vi "WaitFor2DBufferExample.vi"() -> ()   [LabVIEW 2012]
doc: "A short program to demonstrate the fundamentals of control and image acquision with the pco.camera series. The program records a sequence of images, with \"live\" updating, until the \"StopRecording\" button is pressed. A subset of recorded images is then read out from the camera RAM. Warning: Limit the number of images read back tfrom the camera RAM to a reasonable number. Images are stored as a three-dimensional array, which can very large. Use ctrl-H for more help on the individual controls and indicators.\n\nCopyright 2004, the Cooke Corporation."
panel:
  out "bClose":bool
  in  "Quit":bool
  in  "ImageNr":i32
  in  "Image":i32
  out "BufNr1":i16
  out "BufNr0":i16
  in  "bUseBuffer1":bool
  in  "bUseBuffer0":bool
  in  "ROIX1":u16=1 min=1
  in  "ROIY1":u16=1 min=1
  in  "ROIY0":u16=1 min=1
  in  "ROIX0":u16=1 min=1
  in  "InterfaceType":u16(ring)=5 items=["IEEE1394 - Firewire", "IEEE1394/Firewire", "Matrox Helios Camera Link", "Silicon Software ME3 Camera Link", "National Instruments Camera Link", "Gigabit Ethernet", "USB", "Reserved", "Reserved", "Reserved", "Generic Camera Link with CLSER.DLL"]
  out "Bits/pixel":u16
  in  "Readout":bool
  in  "Record":bool
  in  "Open StructureIn":T1={"Size"=88, "InterfaceType"=0, "Camera Number"=0, "CameraNumAtInterface"=0, "OpenFlags"=[], "OpenDWFlags"=[], "OpenPtrs"=[]}
  in  "Stop":u32=10 min=1
  in  "Start":u32=1 min=1
  in  "DelayTimeBase":u16(ring)=2 items=["nanoseconds", "microseconds", "milliseconds"]
  in  "ExposureTimeBase":u16(ring)=2 items=["nanoseconds", "microseconds", "milliseconds"]
  in  "Exposure":u32=10
  in  "Delay":u32
  out "Reading":bool
  in  "StorageMode":bool
  out "ImageCount":u32
  in  "Rate":i32
  out "Image":u16[][](graph)
  in  "TriggerMode":u16(ring) items=["Auto", "Software", "External sequence start ", "External exposure control"]
  # "A short program to demonstrate the fundamentals of control and image acquision with the pco.camera series. The program records a sequence of images, with \"live\" updating, until the \"StopRecording\" button is pressed. A subset of recorded images is then read out from the camera RAM. WARNING: Limit the number of images read back tfrom the camera RAM to a reasonable number. Images are stored as a three-dimensional array, which can very large.  Use ctrl-H for more help on the individual controls and indicators."
  # "pco.labview"
  # "1) Setup camera:"
  # "FIFO"
  # "Recorder"
  # "2) Record  images:"
  # "3) Read out images:"
  # "4) Display image:"
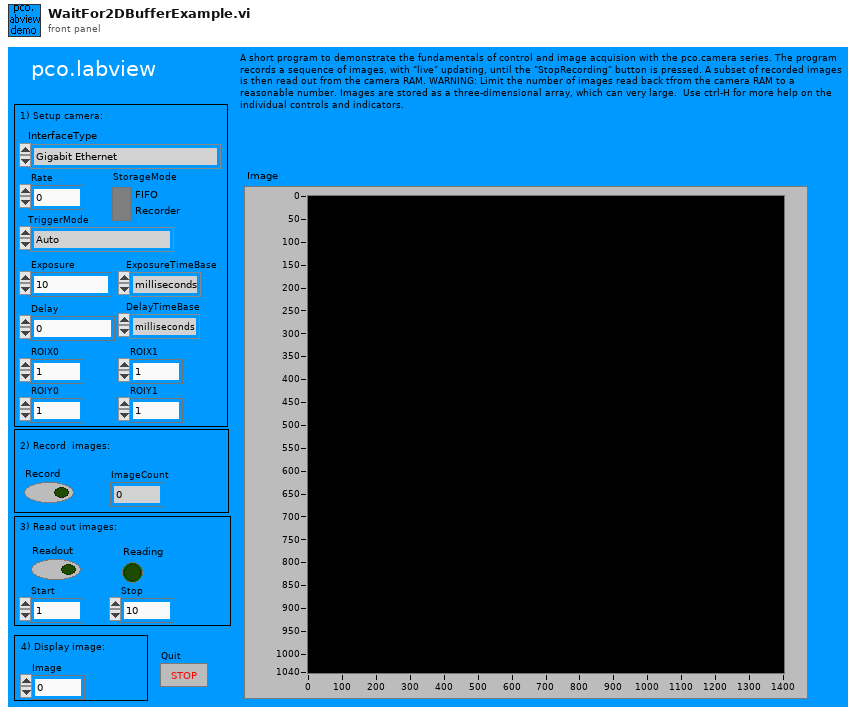
[diagram p1: front panel]
types:
  T1 = cluster{"Size":u16, "InterfaceType":u16, "Camera Number":u16, "CameraNumAtInterface":u16, "OpenFlags":u16[], "OpenDWFlags":u32[], "OpenPtrs":u32[]}
  T2 = cluster{"Size":u16, "CamType":u16, "CamSubType":u16, "SerialNumber":u32, "HWVersion":u32, "FWVersion":u32, "InterfaceType":u16, "HardwareVersion":cluster{"BoardNum":u16, "HWVersions":cluster{"BoardName":string, "BatchNumber":u16, "MinorRevision":u8, "MajorRevision":u8, "Variant":u16}[]}, "FirmwareVersion":cluster{"DeviceNum":u16, "FWVersions":cluster{"DeviceName":string, "MinorRevision":u8, "MajorRevision":u8, "Variant":u16}[]}}
  T3 = cluster{"Size":u16, "SensorTypeDESC":u16, "SensorSubtypeDESC":u16, "MaxHorizontalResStdDESC":u16, "MaxVerticalResStdDESC":u16, "MaxHorizontalResExtDESC":u16, "MaxVerticalResExtDESC":u16, "DynResDESC":u16, "MaxBinHorzDESC":u16, "BinHorzStepDESC":bool, "MaxBinVertDESC":u16, "BinVertStepDESC":bool, "ROIHorzStepDESC":u16, "ROIVertStepDESC":u16, "NumADCDESC":u16, "IRDESC":bool, "MinDelayDESC":u32, "MaxDelayDESC":u32, "MinDelayStepDESC":u32, "MinExpoDESC":u32, "MaxExpoDESC":u32, "MinExpoStepDESC":u32, "MinDelayIRDESC":u32, "MaxDelayIRDESC":u32, "MinExpoIRDESC":u32, "MaxExpoIRDESC":u32, "TimeTableDESC":bool, "DoubleImageDESC":bool, "MinCoolSetDESC":i16, "MaxCoolSetDESC":i16, "MDefaultCoolSetDESC":i16, "PowerDownModeDESC":bool, "OffsetRegDESC":bool, "ColorPattern":cluster{"UpperLeftColor":u8, "UpperRightColor":u8, "LowerLeftColor":u8, "LowerRightColor":u8}, "PatternTypeDESC":bool, "PixelRates":u32[], "CoversionFactors":u16[], "Reserved":u32[], "NoiseFilterCapable":bool, "HotPixelCapable":bool, "HotPixelWithNoiseFilter":bool, "ASCIITimeCapable":bool, "Extended Description":bool, "Get Extended":bool, "Reserved Flag 1":bool, "Reserved Flag 2":bool}
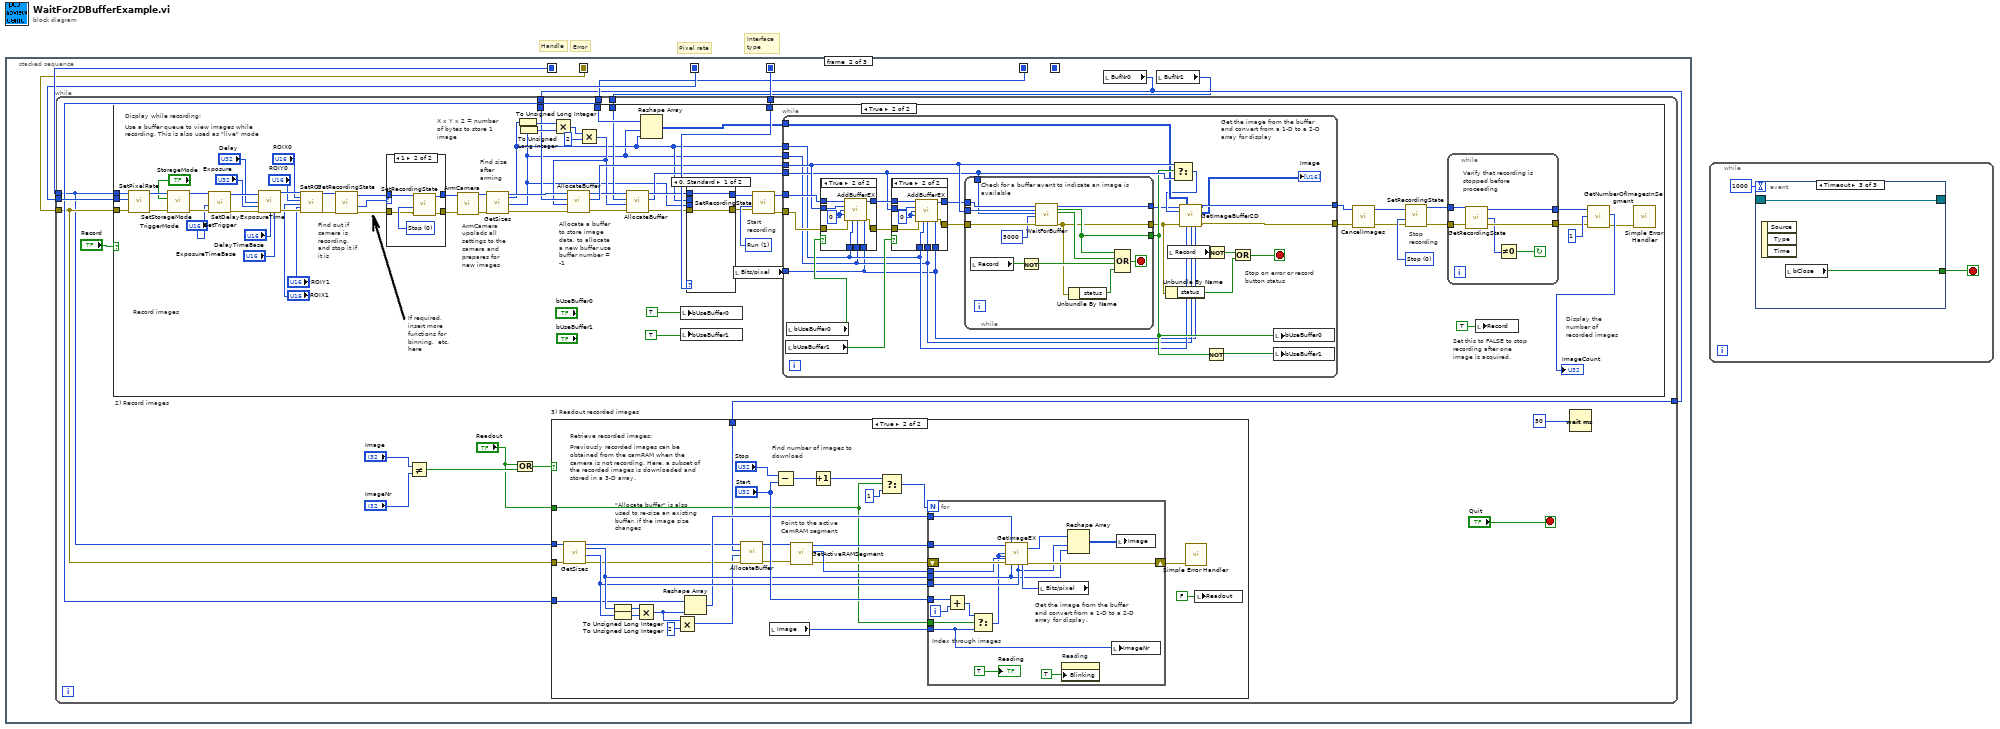
[diagram p0: block diagram]
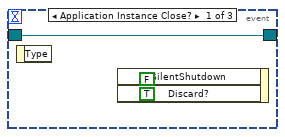
[diagram p2: hidden frame]
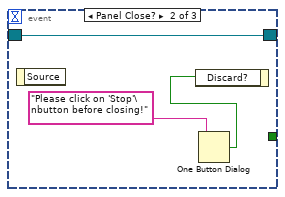
[diagram p3: hidden frame]
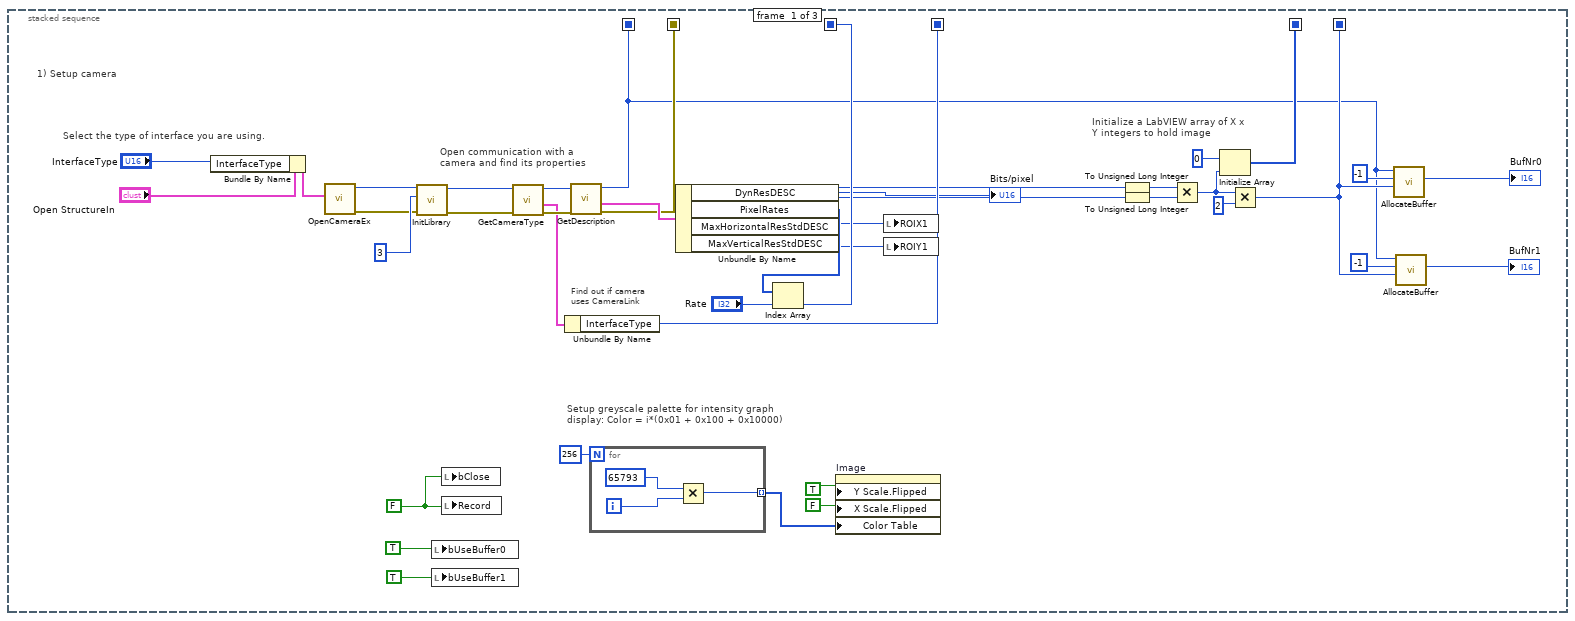
[diagram p4: hidden frame]
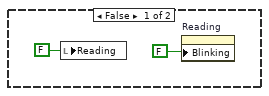
[diagram p5: hidden frame]
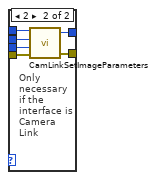
[diagram p9: hidden frame]
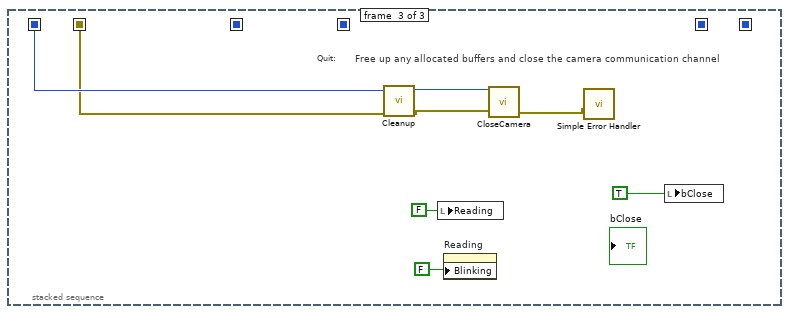
[diagram p11: hidden frame]
diagram:
  # "Interface type"
  # "Error"
  # "Handle"
  # "Pixel rate"
  n1 = stacked-sequence {
    seq-local: [w33 _ _] -> [_ w45 _]
    seq-local: [w13 _ _] -> [_ _ _]
    seq-local: [w25 _ _] -> [_ w47 _]
    seq-local: [w12 _ _] -> [_ w49 w269]
    seq-local: [w24 _ _] -> [_ w48 w268]
    seq-local: [w23 _ _] -> [_ w46 _]
    frame #0 {
      w6 = FALSE ("stop")
      # "Select the type of interface you are using."
      # "1) Setup camera"
      # "Find out if camera uses CameraLink"
      # "Setup greyscale palette for intensity graph display: Color = i*(0x01 + 0x100 + 0x10000)"
      # "Initialize a LabVIEW array of X x Y integers to hold image"
      # "Open communication with a camera and find its properties"
      n2 = Bundle By Name(cluster="Open StructureIn", "InterfaceType"="InterfaceType") -> (w20:T1)
      n3 = call "OpenCameraEx.vi"("OpenStructureIn"=w20) -> ("error out"=w3:errorcluster, "hout"=w4:u64)  [unwired: 3 in, 2 out]
      n4 = call "InitLibrary.vi"("error in (no error)"=w3, "InterfaceType"=u32 3, "ph"=w4) -> ("error out"=w1:errorcluster, "hout"=w2:u64)  [unwired: 7 in]
      n5 = local write "bUseBuffer0"(TRUE) -> ()
      n6 = local write "bUseBuffer1"(TRUE) -> ()
      n7 = local write "bClose"(w6) -> ()
      n8 = local write "Record"(w6) -> ()
      n9 = call "GetCameraType.vi"("ph"=w2, "error in (no error)"=w1) -> ("hout"=w29:u64, "CameraType"=w27:T2, "error out"=w28:errorcluster)  [unwired: 1 in, 1 out]
      n10 = Unbundle By Name(w27) -> ("InterfaceType"=w23:u16)
      n11 = call "GetDescription.vi"("ErrorIn"=w28, "ph"=w29) -> ("ErrorOut"=w24:errorcluster, "Description"=w32:T3, "hout"=w12:u64)  [unwired: 2 in, 1 out]
      n12 = for {
        N: 256 -> [_]
        tunnel: [w40] -> w36 mode=indexing
        i -> [w41]
        n13 = Multiply(x=65793, y=w41) -> (x*y=w40:i32)
      }
      n14 = Unbundle By Name(w32) -> ("DynResDESC"=→"Bits/pixel":u16, "PixelRates"=w26:u32[], "MaxHorizontalResStdDESC"=w18:u16, "MaxVerticalResStdDESC"=w17:u16)
      n15 = Index Array(array=w26, index="Rate") -> (element=w25:u32)
      n16 = property on="Image" class="IntGraph (strikt)"("Y Scale.Flipped"=TRUE, "X Scale.Flipped"=FALSE, "Color Table"=w36) -> ()  [unwired: 2 in, 2 out]
      n17 = local write "ROIX1"(w18) -> ()
      n18 = local write "ROIY1"(w17) -> ()
      n19 = To Unsigned Long Integer(number=w18) -> (unsigned 32bit integer=w15:u32)
      n20 = To Unsigned Long Integer(number=w17) -> (unsigned 32bit integer=w14:u32)
      n21 = Multiply(x=w15, y=w14) -> (x*y=w34:u32)
      n22 = Initialize Array(u16 0 ("Element Data"), w34) -> (w33:u16[])
      n23 = Multiply(x=w34, y=u32 2) -> (x*y=w13:u32)
      n24 = call "AllocateBuffer.vi"("Size"=w13, "BufNr"=i16 -1, "ph"=w12) -> ("BufNrOut"=→"BufNr0":i16)  [unwired: 3 in, 5 out]
      n25 = call "AllocateBuffer.vi"("Size"=w13, "BufNr"=-1, "ph"=w12) -> ("BufNrOut"=→"BufNr1":i16)  [unwired: 3 in, 5 out]
    }
    frame #1 {
      n26 = local read "BufNr0"() -> (w44:i16)
      n27 = local read "BufNr1"() -> (w43:i16)
      n28 = while {
        tunnel: w44 -> [w58]
        tunnel: w44 -> [w59]
        tunnel: w45 -> [w61]
        tunnel: w46 -> [w62]
        tunnel: w47 -> [w63]
        tunnel: w48 -> [w60]
        tunnel: w49 -> [w56]
        tunnel: w43 -> [w57]
        stop <- "Quit" stop-if-true
        n29 = case "2) Record images" shown="True" "Record" {
          tunnel: w56 -> [_ w158]
          tunnel: w60 -> [_ w157]
          tunnel: w63 -> [_ w155]
          tunnel: w62 -> [_ w154]
          tunnel: w61 -> [_ w152]
          tunnel: w59 -> [_ w137]
          tunnel: w57 -> [_ w131]
          frame False {
          }
          frame True {
            w182 = u16 1 items=["Stop", "Run"] ("RecordingState")
            w185 = u16 0 items=["Stop", "Run"] ("RecordingState")
            # "Set this to FALSE to stop recording after one image is acquired."
            # "Display the number of recorded images"
            # "Record images"
            # "Start recording"
            # "Allocate a buffer to store image data. to allocate a new buffer use buffer number = -1"
            # "Find size after arming"
            # "ArmCamera upolads all settings to the camera and prepares for new images"
            # "Find out if camera is recording, and stop it if it is"
            # "If required, insert more functions for binning.  etc. here"
            # "X x Y x 2 = number of bytes to store 1 image"
            # "Stop recording"
            # "Use a buffer queue to view images while recording. This is also used as \"live\" mode"
            # "Display while recording:"
            n30 = call "SetPixelRate.vi"("error in (no error)"=w157, "PixelRate"=w155, "ph"=w158) -> ("error out"=w180:errorcluster, "hout"=w181:u64)  [unwired: 2 in, 1 out]
            n31 = call "SetStorageMode.vi"("error in (no error)"=w180, "StorageMode"="StorageMode", "ph"=w181) -> ("error out"=w172:errorcluster, "hout"=w173:u64)  [unwired: 2 in, 1 out]
            n32 = call "SetTrigger.vi"("error in (no error)"=w172, "TriggerMode"="TriggerMode", "ph"=w173) -> ("error out"=w165:errorcluster, "hout"=w166:u64)  [unwired: 2 in, 1 out]
            n33 = call "SetDelayExposureTime.vi"("ph"=w166, "Delay"="Delay", "Exposure"="Exposure", "error in (no error)"=w165, "DelayTimeBase"="DelayTimeBase", "ExposureTimeBase"="ExposureTimeBase") -> ("hout"=w145:u64, "error out"=w143:errorcluster)  [unwired: 7 in, 1 out]
            n34 = call "SetROI.vi"("ph"=w145, "ROIX0"="ROIX0", "ROIY0"="ROIY0", "ROIX1"="ROIX1", "ROIY1"="ROIY1", "error in (no error)"=w143) -> ("hout"=w144:u64, "error out"=w142:errorcluster)  [unwired: 12 in]
            n35 = call "GetRecordingState.vi"("ErrorIn"=w142, "ph"=w144) -> ("ErrorOut"=w176:errorcluster, "RecordingState"=w178:u16, "hout"=w177:u64)  [unwired: 2 in, 1 out]
            n36 = case shown="1" w178 {
              tunnel: w177 -> [w262 w266]
              tunnel: w176 -> [w261 w265]
              tunnel: [w262 w264] -> w175
              tunnel: [w261 w263] -> w174
              frame 0, Default {
              }
              frame 1 {
                w267 = u16 0 items=["Stop", "Run"] ("RecordingState")
                n37 = call "SetRecordingState.vi"("ErrorIn"=w265, "RecordingState"=w267, "ph"=w266) -> ("ErrorOut"=w263:errorcluster, "hout"=w264:u64)  [unwired: 2 in, 1 out]
              }
            }
            n38 = call "ArmCamera.vi"("error in (no error)"=w174, "ph"=w175) -> ("error out"=w170:errorcluster, "hout"=w171:u64)  [unwired: 1 in, 1 out]
            n39 = call "GetSizes.vi"("ph"=w171, "ErrorIn"=w170) -> ("hout"=w167:u64, "XResAct"=w116:u16, "YResAct"=w115:u16, "ErrorOut"=w169:errorcluster)  [unwired: 11 in, 3 out]
            n40 = To Unsigned Long Integer(number=w116) -> (unsigned 32bit integer=w146:u32)
            n41 = To Unsigned Long Integer(number=w115) -> (unsigned 32bit integer=w147:u32)
            n42 = Multiply(x=w146, y=w147) -> (x*y=w148:u32)
            n43 = Multiply(x=w148, y=u32 2) -> (x*y=w132:u32)
            n44 = call "AllocateBuffer.vi"("error in (no error)"=w169, "Size"=w132, "BufNr"=w137, "ph"=w167) -> ("error out"=w136:errorcluster, "BufNrOut"=w149:i16, "hout"=w134:u64)  [unwired: 2 in, 3 out]
            n45 = call "AllocateBuffer.vi"("error in (no error)"=w136, "Size"=w132, "BufNr"=w131, "ph"=w134) -> ("error out"=w135:errorcluster, "BufNrOut"=w130:i16, "hout"=w133:u64)  [unwired: 2 in, 3 out]
            n46 = Reshape Array(w152, w115, w116) -> (w151:u16[][])
            n47 = local write "bUseBuffer0"(TRUE) -> ()
            n48 = local write "bUseBuffer1"(TRUE) -> ()
            n49 = case shown="0, Standard" w154 {
              tunnel: w135 -> [w253 w260]
              tunnel: [w253 w259] -> w160
              tunnel: w133 -> [w254 w258]
              tunnel: [w254 w257] -> w159
              tunnel: w115 -> [_ w256]
              tunnel: w116 -> [_ w255]
              frame 0, Default {
              }
              frame 2 {
                # "Only necessary if the interface is Camera Link"
                n50 = call "CamLinkSetImageParameters.vi"("error in (no error)"=w260, "YRes"=w256, "XRes"=w255, "ph"=w258) -> ("error out"=w259:errorcluster, "hout"=w257:u64)  [unwired: 1 out]
              }
            }
            n51 = local read "Bits/pixel"() -> (w123:u16)
            n52 = call "SetRecordingState.vi"("ErrorIn"=w160, "RecordingState"=w182, "ph"=w159) -> ("ErrorOut"=w156:errorcluster, "hout"=w153:u64)  [unwired: 2 in, 1 out]
            n53 = while {
              tunnel: w149 -> [w203]
              tunnel: w151 -> [w192]
              tunnel: w153 -> [w210]
              tunnel: w115 -> [w194]
              tunnel: w116 -> [w195]
              tunnel: w156 -> [w208]
              tunnel: [w188] -> w122
              tunnel: [w187] -> w121
              tunnel: w130 -> [w202]
              tunnel: w123 -> [w193]
              stop <- w196 stop-if-true
              # "Stop on error or record button status"
              # "Get the image from the buffer and convert from a 1-D to a 2-D array for display"
              n54 = local read "bUseBuffer1"() -> (w205:bool)
              n55 = local read "bUseBuffer0"() -> (w206:bool)
              n56 = case shown="True" w206 {
                tunnel: [w213 w222] -> w207
                tunnel: [w212 w221] -> w209
                tunnel: w203 -> [_ w220]
                tunnel: w210 -> [w212 w219]
                tunnel: w193 -> [_ w217]
                tunnel: w195 -> [_ w216]
                tunnel: w194 -> [_ w215]
                tunnel: w208 -> [w213 w214]
                frame False {
                }
                frame True {
                  w218 = 0
                  n57 = call "AddBufferEX.vi"("ph"=w219, "BuffNr"=w220, "1stImage"=w218, "LastImage"=w218, "error in (no error)"=w214, "XRes"=w216, "YRes"=w215, "BitPerPixel"=w217) -> ("hout"=w221:u64, "error out"=w222:errorcluster)  [unwired: 5 in, 1 out]
                }
              }
              n58 = case shown="True" w205 {
                tunnel: [w223 w233] -> w200
                tunnel: [w224 w232] -> w201
                tunnel: w202 -> [_ w231]
                tunnel: w209 -> [w224 w230]
                tunnel: w193 -> [_ w228]
                tunnel: w195 -> [_ w227]
                tunnel: w194 -> [_ w226]
                tunnel: w207 -> [w223 w225]
                frame False {
                }
                frame True {
                  w229 = 0
                  n59 = call "AddBufferEX.vi"("ph"=w230, "BuffNr"=w231, "1stImage"=w229, "LastImage"=w229, "error in (no error)"=w225, "XRes"=w227, "YRes"=w226, "BitPerPixel"=w228) -> ("hout"=w232:u64, "error out"=w233:errorcluster)  [unwired: 5 in, 1 out]
                }
              }
              n60 = while {
                tunnel: w203 -> [w241]
                tunnel: w202 -> [w240]
                tunnel: w201 -> [w243]
                tunnel: w200 -> [w242]
                tunnel: [w239] -> w190
                tunnel: [w235] -> w189
                tunnel: [w238] -> w199
                stop <- w244 stop-if-true
                # "Check for a buffer event to indicate an image is available"
                n61 = local read "Record"() -> (w246:bool)
                n62 = Not(x=w246) -> (.not. x?=w245:bool)
                n63 = call "WaitForBuffer.vi"("ph"=w243, "sBufNr"=w241, "sBufNr 2"=w240, "timeout"=5000, "error in (no error)"=w242) -> ("hout"=w239:u64, "Buffer_Ready"=w238:bool, "Buffer_Ready 2"=w237:bool, "error out"=w235:errorcluster)  [unwired: 10 in, 1 out]
                n64 = Unbundle By Name(w235) -> ("status"=w234:bool)
                n65 = Compound Arithmetic op=OR(w238, w237, w245, w234) -> (w244:bool)
              }
              n66 = Unbundle By Name(w189) -> ("status"=w197:bool)
              n67 = local read "Record"() -> (w211:bool)
              n68 = Select(t=w203, s=w199, f=w202) -> (s? t:f=w191:i16)
              n69 = call "GetImageBuffer2D.vi"("ph"=w190, "BuffIn"=w192, "BuffNr"=w191, "error in (no error)"=w189, "xRes"=w195, "yRes"=w194, "Bitresolution"=w193) -> ("hout"=w188:u64, "BuffOut"=→"Image":u16[][], "error out"=w187:errorcluster)  [unwired: 5 in, 1 out]
              n70 = Not(x=w199) -> (.not. x?=w204:bool)
              n71 = Not(x=w211) -> (.not. x?=w198:bool)
              n72 = Or(x=w198, y=w197) -> (x .or. y?=w196:bool)
              n73 = local write "bUseBuffer0"(w199) -> ()
              n74 = local write "bUseBuffer1"(w204) -> ()
            }
            n75 = call "CancelImages.vi"("error in (no error)"=w121, "ph"=w122) -> ("error out"=w127:errorcluster, "hout"=w126:u64)  [unwired: 1 in, 1 out]
            n76 = call "SetRecordingState.vi"("ErrorIn"=w127, "RecordingState"=w185, "ph"=w126) -> ("ErrorOut"=w183:errorcluster, "hout"=w184:u64)  [unwired: 2 in, 1 out]
            n77 = while {
              tunnel: [w250] -> w120
              tunnel: w183 -> [w251]
              tunnel: w184 -> [w252]
              tunnel: [w247] -> w119
              stop <- w248 continue-if-true
              # "Verify that recording is stopped before proceeding"
              n78 = call "GetRecordingState.vi"("ErrorIn"=w251, "ph"=w252) -> ("ErrorOut"=w250:errorcluster, "RecordingState"=w249:u16, "hout"=w247:u64)  [unwired: 2 in, 1 out]
              n79 = Not Equal To 0?(x=w249) -> (x != 0?=w248:bool)
            }
            n80 = local write "Record"(TRUE ("Record")) -> ()
            n81 = call "GetNumberOfImagesInSegment.vi"("ph"=w119, "Segment"=u16 1, "error in (no error)"=w120) -> ("ValidImageCnt"=→"ImageCount":u32, "error out"=w118:errorcluster)  [unwired: 3 out]
            n82 = call <vilib>:"Simple Error Handler.vi"("error in (no error)"=w118) -> ()  [unwired: 4 in, 5 out]
          }
        }
        n83 = Not Equal?(x="Image", y="ImageNr") -> (x != y?=w53:bool)
        n84 = Or(x="Readout", y=w53) -> (x .or. y?=w52:bool)
        n85 = case "3) Readout recorded images" shown="True" w52 {
          tunnel: w61 -> [_ w89]
          tunnel: w56 -> [_ w81]
          tunnel: w60 -> [_ w80]
          tunnel: w58 -> [_ w74]
          tunnel: "Readout" -> [_ w68]
          frame False {
            n86 = local write "Reading"(FALSE ("Reading")) -> ()
            n87 = property on="Reading" class="Bool. (strikt)"("Blinking"=FALSE) -> ()  [unwired: 2 in, 2 out]
          }
          frame True {
            # "Point to the active CamRAM segment"
            # "\"Allocate buffer\" is also used to re-size an existing buffer, if the image size changes"
            # "Find number of images to download"
            # "Previously recorded images can be obtained from the camRAM when the camera is not recording. Here, a subset of the recorded images is downloaded and stored in a 3-D array."
            # "Retrieve recorded images:"
            n88 = call "GetSizes.vi"("ph"=w81, "ErrorIn"=w80) -> ("hout"=w87:u64, "XResAct"=w91:u16, "YResAct"=w90:u16, "ErrorOut"=w85:errorcluster)  [unwired: 11 in, 3 out]
            n89 = To Unsigned Long Integer(number=w91) -> (unsigned 32bit integer=w77:u32)
            n90 = To Unsigned Long Integer(number=w90) -> (unsigned 32bit integer=w78:u32)
            n91 = Multiply(x=w77, y=w78) -> (x*y=w79:u32)
            n92 = Multiply(x=w79, y=u32 2) -> (x*y=w76:u32)
            n93 = Reshape Array(w89, w79) -> (w88:u16[])
            n94 = call "AllocateBuffer.vi"("error in (no error)"=w85, "Size"=w76, "BufNr"=w74, "ph"=w87) -> ("error out"=w84:errorcluster, "hout"=w86:u64)  [unwired: 2 in, 4 out]
            n95 = local read "Image"() -> (w72:i32)
            n96 = Subtract(x="Stop", y="Start") -> (x-y=w95:u32)
            n97 = call "GetActiveRAMSegment.vi"("error in (no error)"=w84, "ph"=w86) -> ("error out"=w82:errorcluster, "ActSeg"=w92:u16, "hout"=w83:u64)  [unwired: 2 in, 1 out]
            n98 = Increment(x=w95) -> (x+1=w71:u32)
            n99 = Select(t=w71, s=w68, f=1) -> (s? t:f=w70:u32)
            n100 = for {
              N: w70 -> [_]
              tunnel: w83 -> [w114]
              shift-right: [w111] -> w73
              shift-left: w82 -> [w110]
              tunnel: "Start" -> [w107]
              tunnel: w92 -> [w105]
              tunnel: w91 -> [w101]
              tunnel: w90 -> [w102]
              tunnel: w88 -> [w103]
              tunnel: w72 -> [w97]
              tunnel: w68 -> [w99]
              i -> [w106]
              # "Get the image from the buffer and convert from a 1-D to a 2-D array for display."
              # "Index through images"
              n101 = Add(x=w107, y=w106) -> (x+y=w98:u32)
              n102 = Select(t=w98, s=w99, f=w97) -> (s? t:f=w100:u32)
              n103 = local read "Bits/pixel"() -> (w104:u16)
              n104 = call "GetImageEX.vi"("ph"=w114, "1stImage"=w100, "lastImage"=w100, "segment"=w105, "error in (no error)"=w110, "BuffIn"=w103, "xRes"=w101, "yRes"=w102, "BitPerPixel"=w104) -> ("BuffOut"=w113:u16[], "error out"=w111:errorcluster)  [unwired: 7 in, 2 out]
              n105 = property on="Reading" class="Bool. (strikt)"("Blinking"=TRUE) -> ()  [unwired: 2 in, 2 out]
              n106 = Reshape Array(w113, w102, w101) -> (w112:u16[][])
              n107 = local write "ImageNr"(w97) -> ()
              n108 = local write "Image"(w112) -> ()
              "Reading" <- TRUE ("Reading")
            }
            n109 = call <vilib>:"Simple Error Handler.vi"("error in (no error)"=w73) -> ()  [unwired: 4 in, 5 out]
            n110 = local write "Readout"(FALSE ("Readout")) -> ()
          }
        }
        n111 = Wait (ms)(milliseconds to wait=u32 50) -> ()  [unwired: 1 out]
      }
    }
    frame #2 {
      # "Free up any allocated buffers and close the camera communication channel"
      # "Quit:"
      n112 = call "Cleanup.vi"("error in (no error)"=w268, "ph"=w269) -> ("error out"=w271:errorcluster, "hout"=w270:u64)  [unwired: 8 in]
      n113 = local write "Reading"(FALSE ("Reading")) -> ()
      n114 = property on="Reading" class="Bool. (strikt)"("Blinking"=FALSE) -> ()  [unwired: 2 in, 2 out]
      n115 = call "CloseCamera.vi"("ErrorIn"=w271, "Handle in"=w270) -> ("ErrorOut"=w273:errorcluster)  [unwired: 1 in, 2 out]
      n116 = call <vilib>:"Simple Error Handler.vi"("error in (no error)"=w273) -> ()  [unwired: 4 in, 5 out]
      n117 = local write "bClose"(TRUE) -> ()
    }
  }
  n118 = while {
    stop <- w276 stop-if-true
    n119 = event shown="[2] Timeout" {
      selector: _ -> [w278 w283 w285]
      dyn-events: [w278 w283 w285] -> _
      timeout: 1000 -> [_ _ _]
      tunnel: [_ _ w284] -> w276
      event Application Instance Close? {
        n120 = event-data() -> ()  [unwired: 1 in, 1 out]
        n121 = event-data("SilentShutdown"=FALSE, "Discard?"=TRUE) -> ()  [unwired: 1 in, 1 out]
      }
      event Panel Close? {
        n122 = event-data() -> ()  [unwired: 1 in, 1 out]
        n123 = One Button Dialog(message="Please click on 'Stop'\nbutton before closing!") -> (true=w281:bool)  [unwired: 1 in]
        n124 = event-data("Discard?"=w281) -> ()  [unwired: 1 in, 1 out]
      }
      event Timeout {
        n125 = event-data() -> ()  [unwired: 1 in, 3 out]
        n126 = local read "bClose"() -> (w284:bool)
      }
    }
  }
